vi "Serial_Setup.vi"() -> ()   [LabVIEW 2011]
uses:
  Port_Params.ctl
  Anemometry/Anemometry Sub Vis/Controls/ok_button.ctl
panel:
  in  "OK":T1
  in  "Port Settings Array":T2[](array[typedef]) {"flow control etc."."parity err byte" format="%.0x"; "flow control etc."."XON byte" format="%.0x"; "flow control etc."."XOFF byte" format="%.0x"; "data bits" min=5 max=8 step=1}
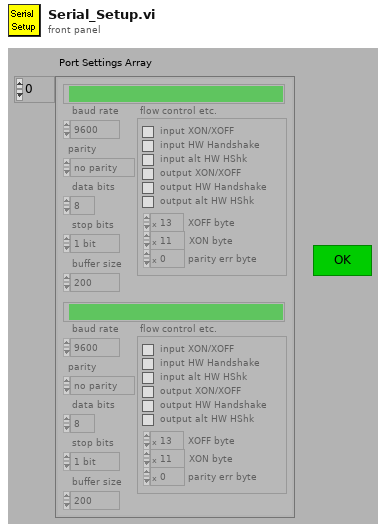
[diagram p1: front panel]
types:
  T1 = typedef "ok_button.ctl" = bool
  T2 = typedef "Port_Params.ctl" = cluster{"Name":string, "flow control etc.":cluster{"input XON/XOFF":bool, "input HW Handshake":bool, "input alt HW HShk":bool, "output XON/XOFF":bool, "output HW Handshake":bool, "output alt HW HShk":bool, "XOFF byte ":u8, "XON byte":u8, "parity err byte":u16}, "buffer size":u16, "baud rate":u32, "data bits":u16, "stop bits":enum16{"1 bit", "1.5 bits", "2 bits"}, "parity":enum16{"no parity", "odd parity", "even parity", "mark parity", "space parity"}}
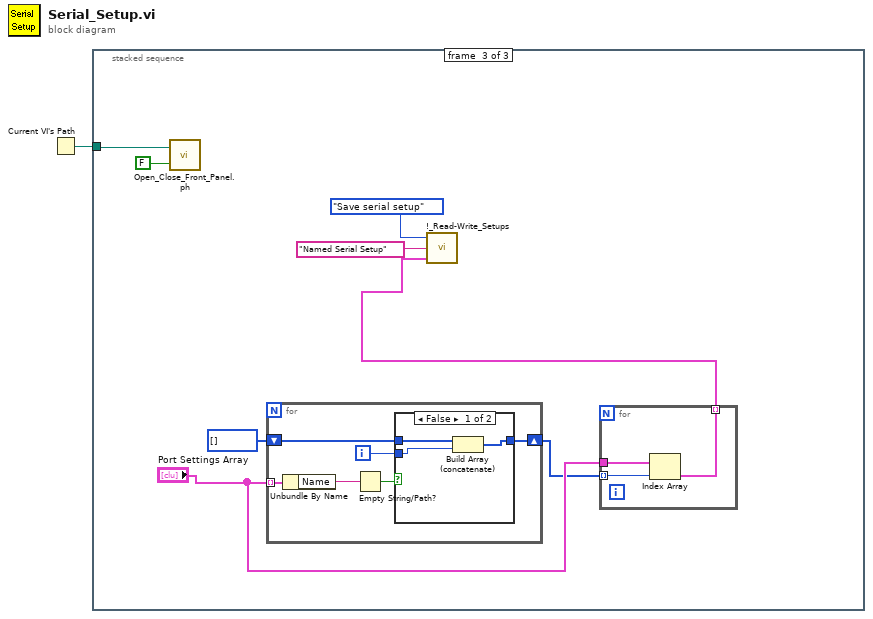
[diagram p0: block diagram]
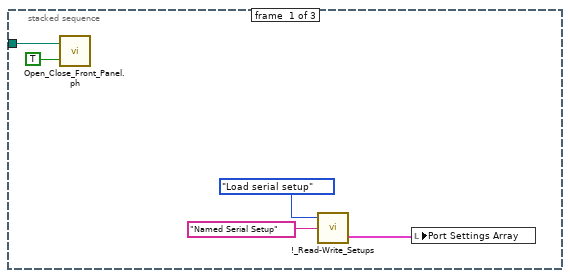
[diagram p2: hidden frame]
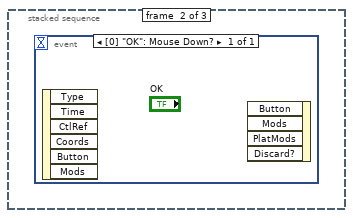
[diagram p3: hidden frame]
diagram:
  n1 = Current VI's Path() -> (path=w1:path)
  n2 = stacked-sequence {
    tunnel: w1 -> [w3 _ w7]
    frame #0 {
      n3 = call "Open_Close_Front_Panel.ph.vi"("Front Panel Window:Open"=TRUE, "VI path"=w3) -> ()  [unwired: 1 in, 1 out]
      n4 = call "!_Read-Write_Setups.vi"("Setup Name"="Named Serial Setup", "Mode"=enum16{"Load serial setup", "Save serial setup"}."Load serial setup") -> ("Port Settings Array Out"=w4:T2[])  [unwired: 1 in, 1 out]
      n5 = local write "Port Settings Array"(w4) -> ()
    }
    frame #1 {
      n6 = event shown="[0] \"OK\": Mouse Down?" {
        selector: _ -> [_]
        dyn-events: _ -> [_]
        timeout: _ -> [_]
        event Mouse Down? {
          n7 = event-data() -> ()  [unwired: 1 in, 6 out]
          n8 = event-data() -> ()  [unwired: 5 in, 1 out]
        }
      }
    }
    frame #2 {
      n9 = call "Open_Close_Front_Panel.ph.vi"("Front Panel Window:Open"=FALSE, "VI path"=w7) -> ()  [unwired: 1 in, 1 out]
      n10 = for {
        shift-right: [w19] -> w10
        shift-left: i32[] [] -> [w20]
        tunnel: "Port Settings Array" -> [w23] mode=indexing
        i -> [w18]
        n11 = Unbundle By Name(w23) -> ("Name"=w21:string)
        n12 = Empty String/Path?(string/path=w21) -> (empty?=w22:bool)
        n13 = case shown="False" w22 {
          tunnel: w20 -> [w25 w27]
          tunnel: [w24 w27] -> w19
          tunnel: w18 -> [w26 _]
          frame False {
            n14 = Build Array (concatenate)(w25, w26) -> (w24:i32[])
          }
          frame True {
          }
        }
      }
      n15 = for {
        tunnel: "Port Settings Array" -> [w17]
        tunnel: w10 -> [w16] mode=indexing
        tunnel: [w15] -> w9 mode=indexing
        n16 = Index Array(array=w17, index=w16) -> (element=w15:T2)
      }
      n17 = call "!_Read-Write_Setups.vi"("Port Settings Array In"=w9, "Setup Name"="Named Serial Setup", "Mode"=enum16{"Load serial setup", "Save serial setup"}."Save serial setup") -> ()  [unwired: 2 out]
    }
  }
